vi "Initialize Session.vi"(5 "Password":string, 6 "Connect Timeout (4000 ms)":u32=4000, 7 "User Name":string, 8 "error in (no error)":errorcluster, 9 "Language (Automatic)":T1 items=["Automatic"=0, "Chinese Simplified"=2052, "English"=1033, "French"=1036, "German"=1031, "Japanese"=1041, "Korean"=1042], 10 "Force Property Refresh (T)":bool=TRUE, 11 "Target (localhost)":refnum<k21>="localhost") -> (0 "error out":errorcluster, 3 "Session out":refnum<k21>)   [LabVIEW 2017, in "nisyscfg.lvlib"]
doc: "Initializes any system configuration VI to gather information from a specified target. You must use this VI to obtain a handle for a specified target that can be used in other System Configuration VIs.\n\n<B>NOTE:</B> This VI communicates to the device at the specified address. If the device is no longer online, but it has previously been discovered in Measurement & Automation Explorer (MAX), this VI succeeds, allowing you to retrieve cached information about the device. To determine if a Real-Time target is online, use the System Property Node to return the System Status property."
uses:
  <vilib>/nisyscfg/nisyscfg.lvlib
  <vilib>/nisyscfg/Language.ctl
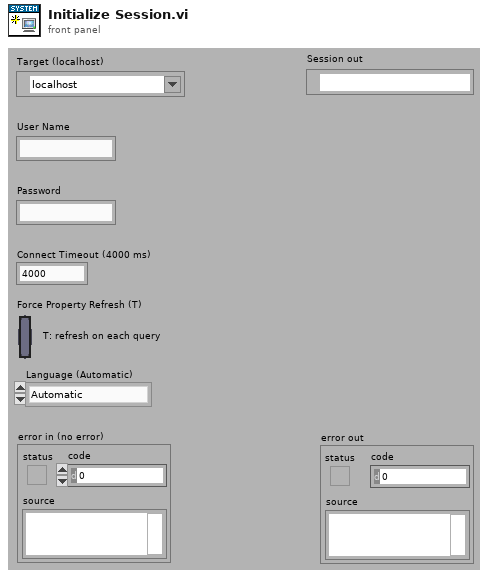
[diagram p1: front panel]
types:
  T1 = typedef "nisyscfg.lvlib/Language.ctl" = i32
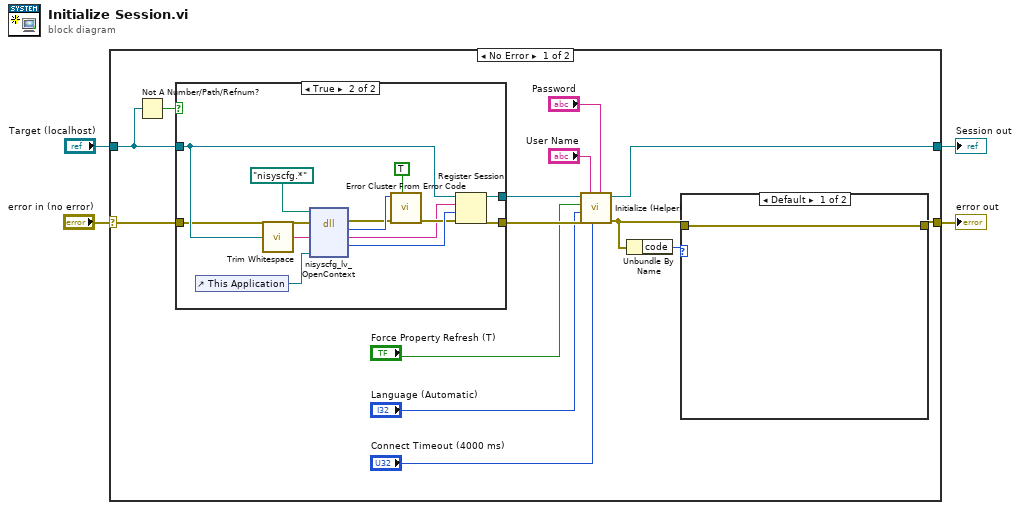
[diagram p0: block diagram]
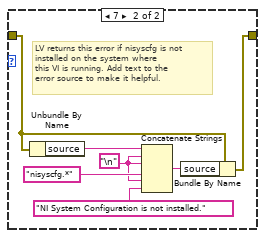
[diagram p2: hidden frame]
diagram:
  n1 = case shown="No Error" "error in (no error)" {
    selector: "error in (no error)" -> [w12 w43]
    tunnel: [w6 w43] -> w4
    tunnel: [w11 w42] -> w2
    tunnel: "Target (localhost)" -> [w17 w42]
    frame No Error {
      n2 = Not A Number/Path/Refnum?(number/path/refnum=w17) -> (NaN/Path/Refnum?=w18:bool)
      n3 = case shown="True" w18 {
        tunnel: w12 -> [w27 w33]
        tunnel: [w27 w41] -> w16
        tunnel: [w28 w40] -> w13
        tunnel: w17 -> [w28 w37]
        frame False {
        }
        frame True {
          n4 = control-ref of="This Application"() -> (w29:refnum<vi>)
          n5 = call <vilib>:"Trim Whitespace.vi"("string"=w37) -> ("trimmed string"=w32:string)  [unwired: 1 in]
          n6 = dll-call lib="nisyscfg.*" fn="nisyscfg_lv_OpenContext" label="OpenContext"(path in=path "nisyscfg.*", error in=w33, "target"=w32, "appReference"=w29) -> (error out=w38:errorcluster, "status"=w39:i32, "target"=w34:string, "sessionHandle"=w36:u64)  [unwired: 1 in, 3 out]
          n7 = call <vilib>:"Error Cluster From Error Code.vi"("show call chain? (False)"=TRUE, "error in (no error)"=w38, "error code (0)"=w39) -> ("error out"=w35:errorcluster)  [unwired: 6 out]
          n8 = Register Session(8:w35, 9:w36, 10:w34, 11:w37) -> (0:w41:errorcluster, 3:w40:refnum<k21>)  [unwired: 1 in]
        }
      }
      n9 = call <vilib>:"Initialize (Helper).vi"("Password"="Password", "Connect Timeout (4000 ms)"="Connect Timeout (4000 ms)", "User Name"="User Name", "error in (no error)"=w16, "Language (Automatic)"="Language (Automatic)", "Force Property Refresh (T)"="Force Property Refresh (T)", "Session in"=w13) -> ("error out"=w7:errorcluster, "Session out"=w11:refnum<k21>)  [unwired: 3 in]
      n10 = Unbundle By Name(w7) -> ("code"=w8:i32)
      n11 = case shown="Default" w8 {
        tunnel: w7 -> [w19 w26]
        tunnel: [w19 w25] -> w6
        frame Default {
        }
        frame 7 {
          w21 = "\n"
          # "LV returns this error if nisyscfg is not\ninstalled on the system where\nthis VI is running. Add text to the\nerror source to make it helpful."
          n12 = Unbundle By Name(w26) -> ("source"=w23:string)
          n13 = Concatenate Strings(w23, w21, w21, "nisyscfg.*", w21, "NI System Configuration is not installed.") -> (w24:string)
          n14 = Bundle By Name(cluster=w26, "source"=w24) -> (w25:errorcluster)
        }
      }
    }
    frame Error {
    }
  }
  "error out" <- w4
  "Session out" <- w2
